vi "InstrumentsReadOut_DP_Ver1.0.vi"(5 "Instruments Configs In 2D array":string[][](table) caption="Instruments Configs", 7 "error in":errorcluster) -> (0 "DataArray":dbl[](array[numeric]), 3 "error out":errorcluster)   [LabVIEW 2012]
doc: "Clear selected GPIB device and initialized selected device\nInstruments Configs In 2D array:\n0: Instrument name\n1: GPIB Address\n2: Initialized CMD\n3: Unit factor\n4: Title name\n5: Read Data CMD\n6: Info"
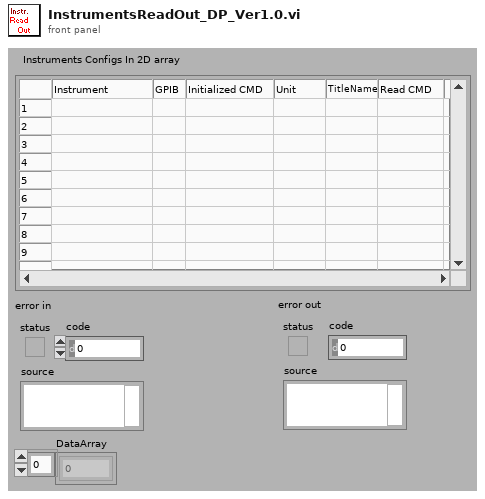
[diagram p1: front panel]
types:
  T1 = enum16{"Instrument", "Function", "GPIB", "Initiralized CMD", "Title Name", "Unit", "Read CMD", "Post CMD", "Info", "Terminator Mode"}
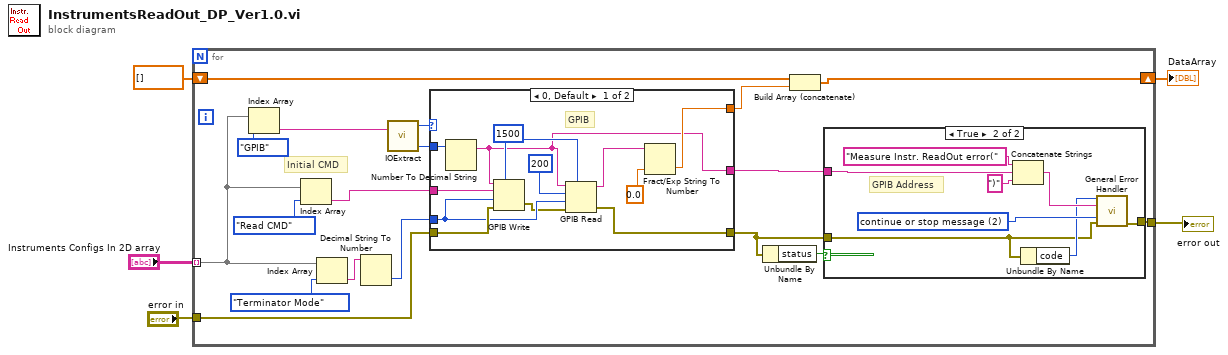
[diagram p0: block diagram]
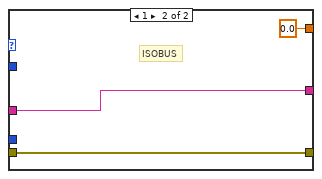
[diagram p2: hidden frame]
diagram:
  n1 = for {
    tunnel: "Instruments Configs In 2D array" -> [w9] mode=indexing
    tunnel: "error in" -> [w15]
    tunnel: [w22] -> w3
    shift-right: [w6] -> w1
    shift-left: dbl[] [] -> [w7]
    # "Initial CMD"
    n2 = Index Array(array=w9, index=T1."GPIB") -> (element=w12:string)
    n3 = Index Array(array=w9, index=T1."Read CMD") -> (element=w17:string)
    n4 = Index Array(array=w9, index=T1."Terminator Mode") -> (element=w18:string)
    n5 = Decimal String To Number(string=w18) -> (number=w16:i32)  [unwired: 2 in, 1 out]
    n6 = call "IOExtract.vi"("Instrument(String)"=w12) -> ("InterfaceCode:\n0: GPIB\n1: ISOBUS"=w11:i32, "Address"=w10:i32)  [unwired: 1 in, 1 out]
    n7 = case shown="0, Default" w11 {
      tunnel: w10 -> [w35 _]
      tunnel: w17 -> [w34 w37]
      tunnel: w16 -> [w31 _]
      tunnel: w15 -> [w33 w38]
      tunnel: [w28 w38] -> w14
      tunnel: [w24 w37] -> w13
      tunnel: [w25 0.0] -> w8
      frame 0, Default {
        w32 = 1500 ("timeout ms (488.2 global)")
        # "GPIB"
        n8 = Number To Decimal String(number=w35) -> (decimal integer string=w24:string)  [unwired: 1 in]
        n9 = GPIB Write(0:w24, 1:w34, 2:w31, 3:w33, 4:w32) -> (6:w30:errorcluster)  [unwired: 1 out]
        n10 = GPIB Read(0:w24, 1:200 ("byte count"), 2:w31, 3:w30, 4:w32) -> (5:w27:string, 7:w28:errorcluster)  [unwired: 1 out]
        n11 = Fract/Exp String To Number(string=w27, default (0 dbl)=0.0) -> (number=w25:dbl)  [unwired: 2 in, 1 out]
      }
      frame 1 {
        # "ISOBUS"
      }
    }
    n12 = Unbundle By Name(w14) -> ("status"=w23:bool)
    n13 = Build Array (concatenate)(w7, w8) -> (w6:dbl[])
    n14 = case shown="True" w23 {
      tunnel: w14 -> [w39 w40]
      tunnel: [w39 w46] -> w22
      tunnel: w13 -> [_ w45]
      frame False {
      }
      frame True {
        w47 = 2 items=["no dialog", "OK message", "continue or stop message"] ("type of dialog (OK msg:1)")
        # "GPIB Address"
        n15 = Concatenate Strings("Measure Instr. ReadOut error(" ("Function"), w45, ")" ("string")) -> (w43:string)
        n16 = Unbundle By Name(w40) -> ("code"=w41:i32)
        n17 = call <vilib>:"General Error Handler.vi"("[error code] (0)"=w41, "[error source] (\" \")"=w43, "type of dialog (OK msg:1)"=w47, "error in (no error)"=w40) -> ("error out"=w46:errorcluster)  [unwired: 7 in, 4 out]
      }
    }
  }
  "error out" <- w3
  "DataArray" <- w1
